vi "Close Device.vi"(8 "error in (no error)":errorcluster, 11 "Device":refnum<class "Device.lvclass">) -> (0 "error out":errorcluster, 3 "Device out":refnum<class "Device.lvclass">)   [LabVIEW 2015, in "Device.lvclass"]
uses:
  Device.lvclass
  Device.lvclass/Device.ctl
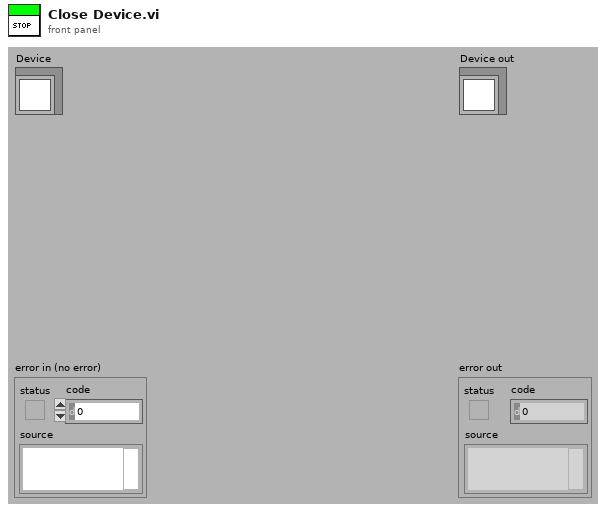
[diagram p1: front panel]
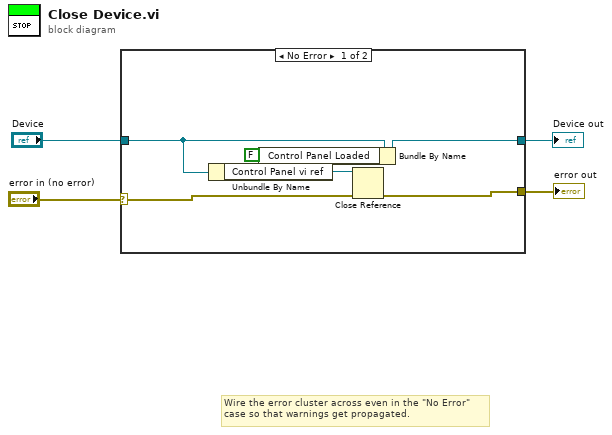
[diagram p0: block diagram]
diagram:
  # "Wire the error cluster across even in the \"No Error\"\ncase so that warnings get propagated."
  n1 = case shown="No Error" "error in (no error)" {
    selector: "error in (no error)" -> [w5 w12]
    tunnel: [w6 w12] -> w3
    tunnel: [w7 w11] -> w1
    tunnel: "Device" -> [w8 w11]
    frame No Error {
      n2 = Unbundle By Name(w8) -> ("Control Panel vi ref"=w10:refnum<vi>)
      n3 = Bundle By Name(cluster=w8, "Control Panel Loaded"=FALSE ("Front Panel Loaded")) -> (w7:refnum<class "Device.lvclass">)
      n4 = Close Reference(reference=w10, error in (no error)=w5) -> (error out=w6:errorcluster)
    }
    frame Error {
    }
  }
  "error out" <- w3
  "Device out" <- w1
